vi "AMI 430_Hardware_Module_X AXIS.vi"(5 "Enable":bool=TRUE, 7 "Command":T4, 8 "error in (no error)":errorcluster, 9 "Settings":T2={"magneticFieldUnits"=1, "rampRateUnits"=1, "rampRate"=0.0, "targetField"=0.0, "rampingMode"=1} {"rampingMode" items=["RAMP", "PAUSE", "MANUAL UP", "MANUAL DOWN", "ZERO"]; "targetField" format="%.4f"; "rampRate" format="%.1f"; "rampRateUnits" items=["Per SECOND", "Per MINUTE"]; "magneticFieldUnits" items=["KGauss", "Tesla"]}, 11 "Comm Config In":T3={"connection ID"=refnum, "IP"="192.168.0.108", "Active Comm Interface"=0, "Serial Port"="", "Programmer Type"=0, "connection ID"=refnum, "output cluster"={"GPIB address"=22, "GPIB bus"=1}} caption="X AXIS: 192.168.0.108" {"Programmer Type" items=["Model 430", "Model 420"]; "Active Comm Interface" items=["TCP/IP (Model 430 Only)", "RS232", "IEEE488"]}) -> (0 "error out":errorcluster, 1 "magneticField":dbl format="%.6f", 2 "Instrument Responded?":bool, 3 "Comm Config Out":T3={"connection ID"=refnum, "IP"="192.168.0.108", "Active Comm Interface"=0, "Serial Port"="", "Programmer Type"=0, "connection ID"=refnum, "output cluster"={"GPIB address"=22, "GPIB bus"=1}} {"Programmer Type" items=["Model 430", "Model 420"]; "Active Comm Interface" items=["TCP/IP (Model 430 Only)", "RS232", "IEEE488"]}, 4 "state":T1=1 items=["Unknown", "RAMPING to target field/current", "HOLDING at the target field/current", "PAUSED", "Ramping in MANUAL UP mode", "Ramping in MANUAL DOWN mode", "ZEROING CURRENT (in progress)", "Quench detected", "At ZERO current", "Heating persistent switch", "Cooling persistent switch", "External Rampdown active"])   [LabVIEW 2017]
uses:
  AMI 430_Hardware_Module.ctl
  commsControl.ctl
  magneticField.ctl
  Status AMI.ctl
panel:
  # "X AXIS"
  # "AMI 430 MAGNETIC FIELD SYSTEM"
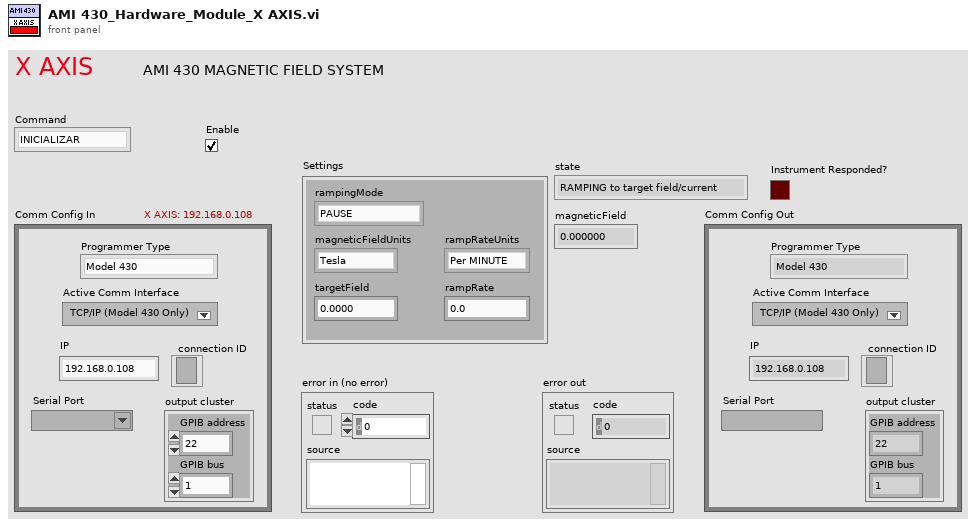
[diagram p1: front panel]
types:
  T1 = typedef "Status AMI.ctl" = u16
  T2 = typedef "magneticField.ctl" = cluster{"magneticFieldUnits":u16, "rampRateUnits":u16, "rampRate":dbl, "targetField":dbl, "rampingMode":u16}
  T3 = typedef "commsControl.ctl" = cluster{"connection ID":refnum<k5>, "IP":string, "Active Comm Interface":u16, "Serial Port":refnum<visa-resource-name>, "Programmer Type":u16, "connection ID":refnum<k5>, "output cluster":cluster{"GPIB address":i16, "GPIB bus":i16}}
  T4 = typedef "AMI 430_Hardware_Module.ctl" = enum16{"INICIALIZAR", "SET UNIDADES CAMPO", "SET UNIDADES RAMPA", "SET CAMPO", "SET  RAMPA", "SET RAMPING MODE", "READ CAMPO", "STATUS", "SHUTDOWN"}
  T5 = cluster{"error":bool, "code":i32, "source":string}
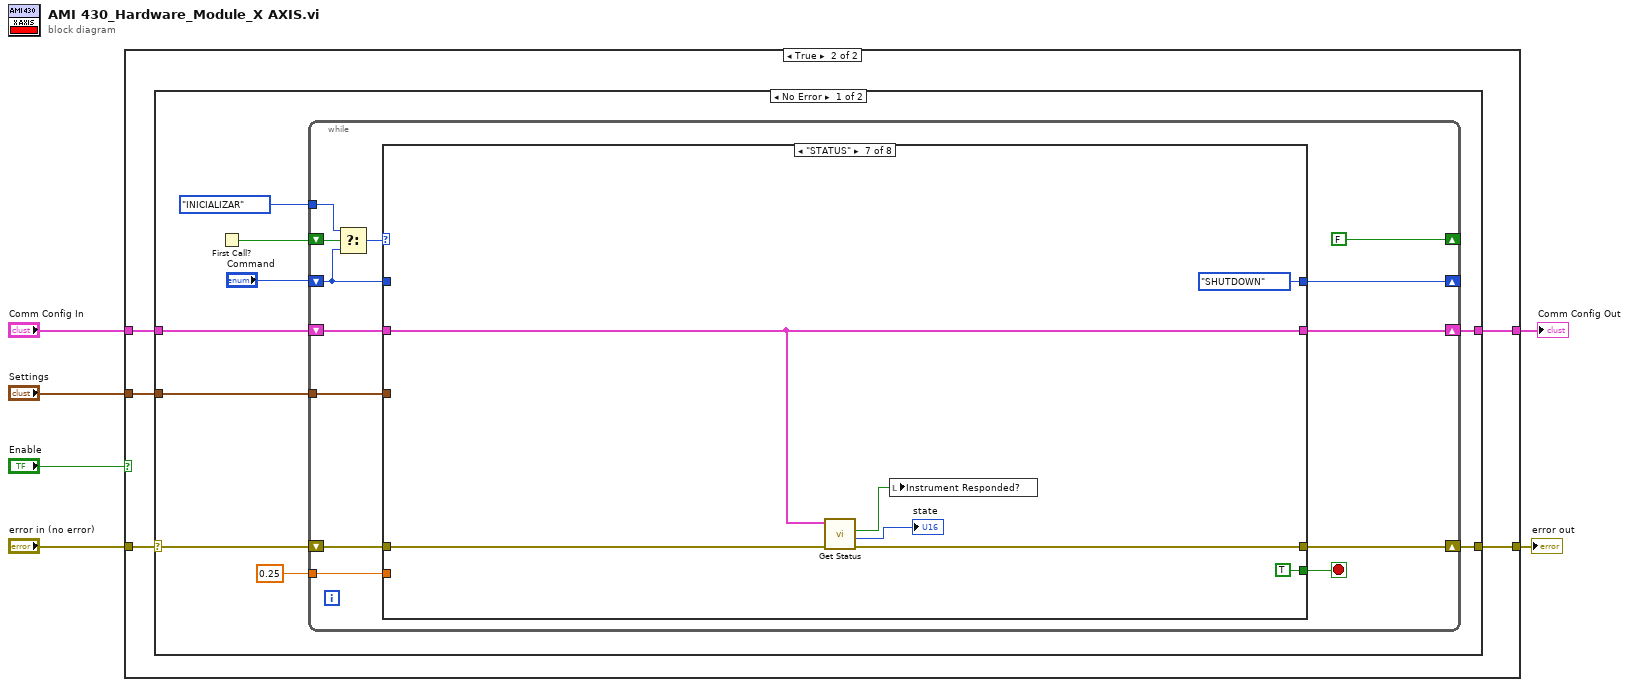
[diagram p0: block diagram]
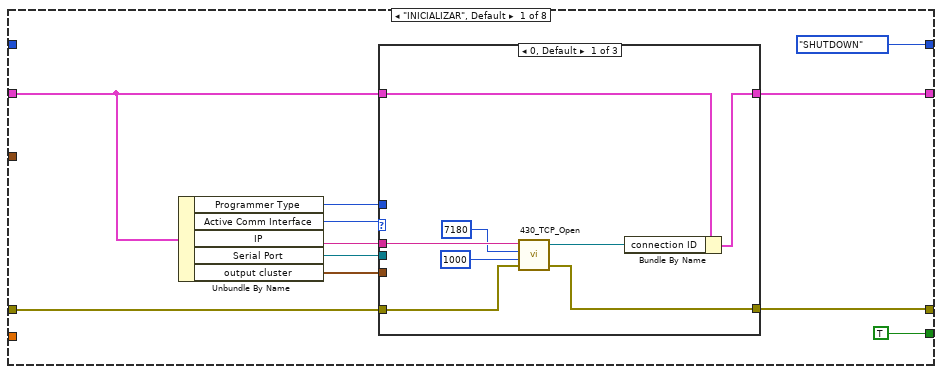
[diagram p3: hidden frame]
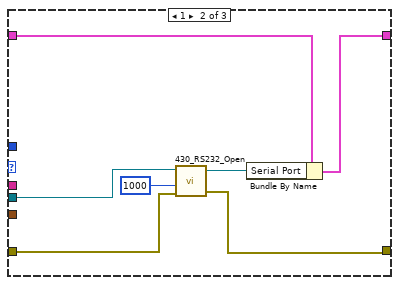
[diagram p4: hidden frame]
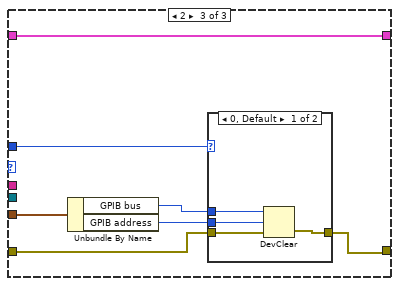
[diagram p5: hidden frame]
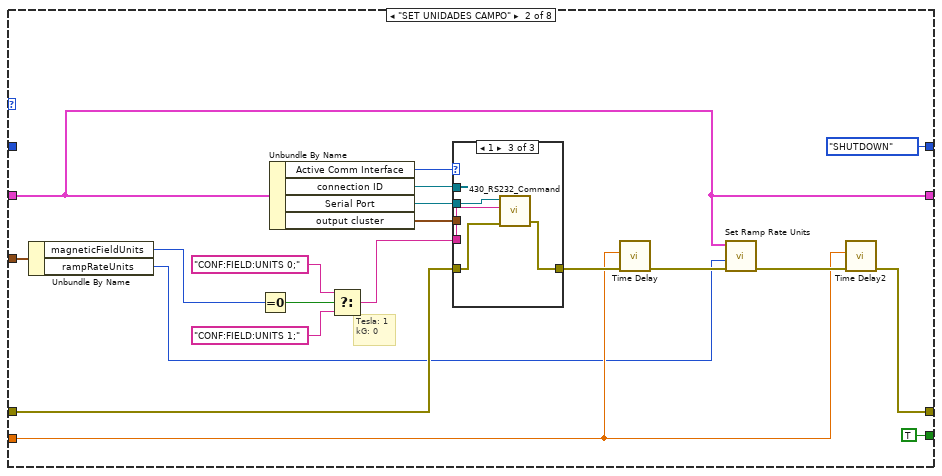
[diagram p7: hidden frame]
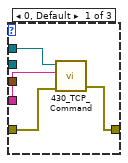
[diagram p8: hidden frame]
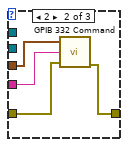
[diagram p9: hidden frame]
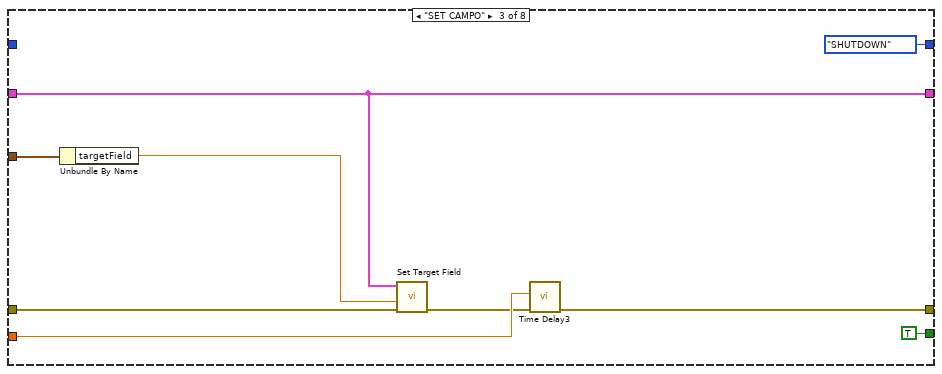
[diagram p10: hidden frame]
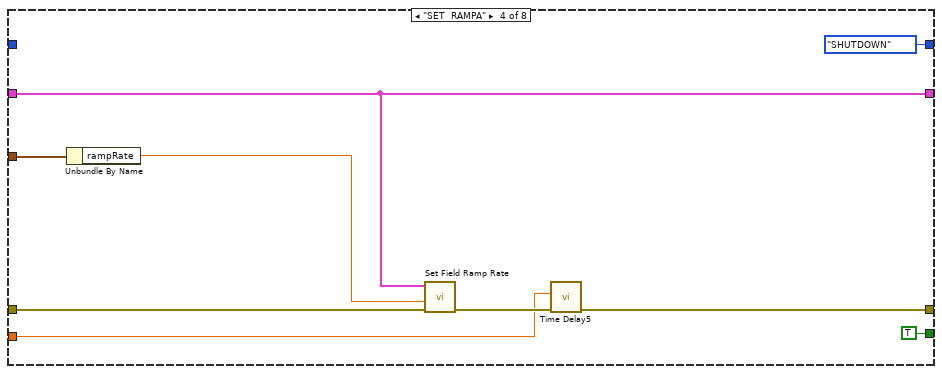
[diagram p11: hidden frame]
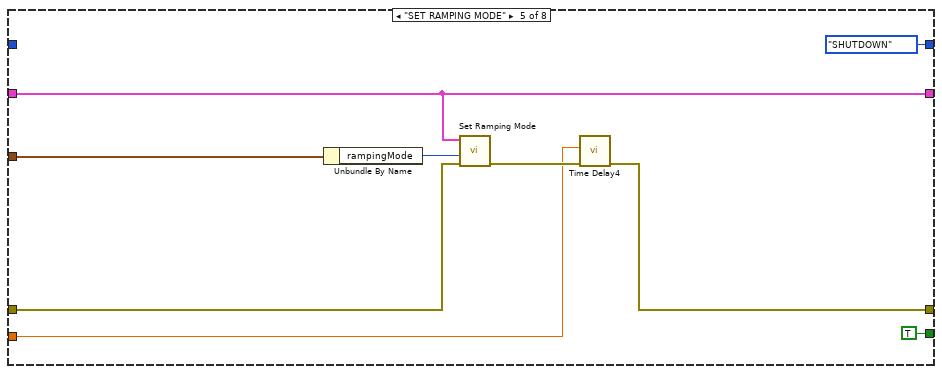
[diagram p12: hidden frame]
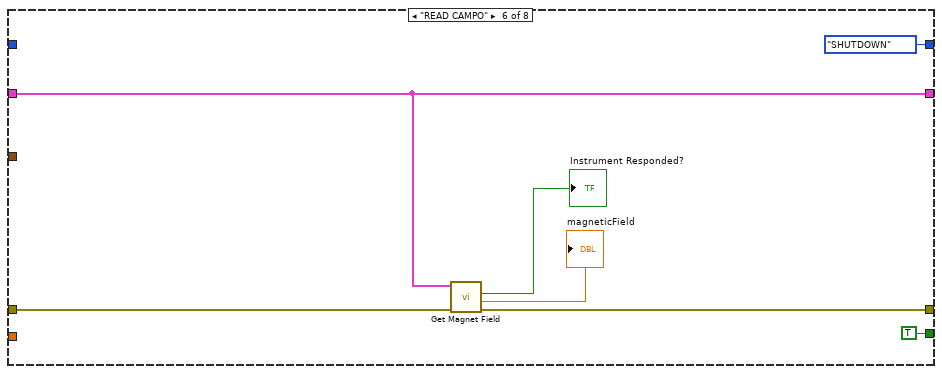
[diagram p13: hidden frame]
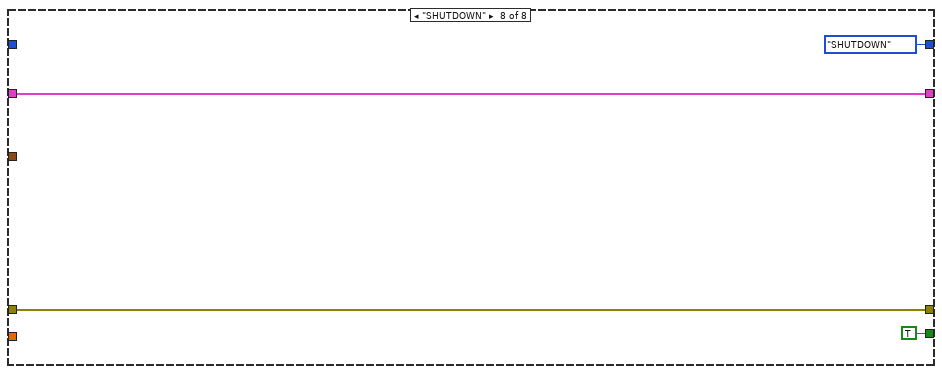
[diagram p14: hidden frame]
diagram:
  n1 = case shown="True" "Enable" {
    tunnel: "error in (no error)" -> [w8 w13]
    tunnel: [w8 w12] -> w5
    tunnel: "Comm Config In" -> [w7 w11]
    tunnel: [w7 w10] -> w2
    tunnel: "Settings" -> [_ w9]
    frame False {
    }
    frame True {
      n2 = case shown="No Error" w13 {
        selector: w13 -> [w20 w152]
        tunnel: [w19 w152] -> w12
        tunnel: w11 -> [w17 w151]
        tunnel: [w16 w151] -> w10
        tunnel: w9 -> [w15 _]
        frame No Error {
          n3 = First Call?() -> (First Call?: T/F=w22:bool)
          n4 = while {
            shift-right: [w30] -> _
            shift-left: "Command" -> [w31]
            shift-right: [w28] -> w19
            shift-left: w20 -> [w26]
            shift-right: [FALSE ("First Call?: T/F")] -> _
            shift-left: w22 -> [w35]
            tunnel: AMI_430_Hardware_Module."INICIALIZAR" ("t") -> [w34]
            shift-right: [w25] -> w16
            shift-left: w17 -> [w27]
            tunnel: w15 -> [w24]
            tunnel: 0.25 ("Delay Time (s)") -> [w23]
            stop <- w29 stop-if-true
            n5 = Select(t=w34, s=w35, f=w31) -> (s? t:f=w32:T4)
            n6 = case shown="\"STATUS\"" w32 {
              tunnel: w31 -> [_ _ _ _ _ _ _ _]
              tunnel: [AMI_430_Hardware_Module."SHUTDOWN" ("s? t:f") AMI_430_Hardware_Module."SHUTDOWN" ("s? t:f") AMI_430_Hardware_Module."SHUTDOWN" ("s? t:f") AMI_430_Hardware_Module."SHUTDOWN" ("s? t:f") AMI_430_Hardware_Module."SHUTDOWN" ("s? t:f") AMI_430_Hardware_Module."SHUTDOWN" ("s? t:f") AMI_430_Hardware_Module."SHUTDOWN" ("s? t:f") AMI_430_Hardware_Module."SHUTDOWN" ("s? t:f")] -> w30
              tunnel: [TRUE ("First Call?: T/F") TRUE ("First Call?: T/F") TRUE ("First Call?: T/F") TRUE ("First Call?: T/F") TRUE ("First Call?: T/F") TRUE ("First Call?: T/F") TRUE ("First Call?: T/F") TRUE ("First Call?: T/F")] -> w29
              tunnel: [w39 w76 w112 w120 w130 w138 w145 w150] -> w28
              tunnel: w27 -> [w38 w87 w109 w117 w125 w135 w142 w147]
              tunnel: [w37 w87 w109 w117 w125 w135 w142 w147] -> w25
              tunnel: w26 -> [w36 w88 w106 w121 w132 w139 w146 w150]
              tunnel: w24 -> [_ w79 w108 w116 w128 _ _ _]
              tunnel: w23 -> [_ w75 w114 w122 w129 _ _ _]
              frame "INICIALIZAR", Default {
                n7 = Unbundle By Name(w38) -> ("Programmer Type"=w40:u16, "Active Comm Interface"=w42:u16, "IP"=w44:string, "Serial Port"=w43:refnum<visa-resource-name>, "output cluster"=w41:cluster{"GPIB address":i16, "GPIB bus":i16})
                n8 = case shown="0, Default" w42 {
                  tunnel: w38 -> [w54 w59 w65]
                  tunnel: w36 -> [w52 w60 w68]
                  tunnel: [w51 w57 w67] -> w39
                  tunnel: w44 -> [w50 _ _]
                  tunnel: [w47 w58 w65] -> w37
                  tunnel: w43 -> [_ w56 _]
                  tunnel: w41 -> [_ _ w64]
                  tunnel: w40 -> [_ _ w66]
                  frame 0, Default {
                    n9 = call "430_TCP_Open.vi"("IP Address"=w50, "TCP Port"=7180, "timeout ms (2000)"=1000 ("timeout ms (60000)"), "error in (no error)"=w52) -> ("connection ID"=w53:refnum<k5>, "error out"=w51:errorcluster)  [unwired: 2 in, 1 out]
                    n10 = Bundle By Name(cluster=w54, "connection ID"=w53) -> (w47:T3)
                  }
                  frame 1 {
                    n11 = call "430_RS232_Open.vi"("VISA resource name"=w56, "timeout ms (2000)"=1000 ("timeout ms (60000)"), "error in (no error)"=w60) -> ("VISA resource name out"=w61:refnum<visa-resource-name>, "error out"=w57:errorcluster)  [unwired: 4 in]
                    n12 = Bundle By Name(cluster=w59, "Serial Port"=w61) -> (w58:T3)
                  }
                  frame 2 {
                    n13 = Unbundle By Name(w64) -> ("GPIB bus"=w63:i16, "GPIB address"=w62:i16)
                    n14 = case shown="0, Default" w66 {
                      tunnel: w68 -> [w72 w73]
                      tunnel: [w71 w73] -> w67
                      tunnel: w63 -> [w70 _]
                      tunnel: w62 -> [w69 _]
                      frame 0, Default {
                        n15 = DevClear(2:w72, 3:w69, 4:w70) -> (0:w71:errorcluster)  [unwired: 1 out]
                      }
                      frame 1 {
                      }
                    }
                  }
                }
              }
              frame "SET UNIDADES CAMPO" {
                # "Tesla: 1\nkG: 0"
                n16 = Unbundle By Name(w79) -> ("magneticFieldUnits"=w78:u16, "rampRateUnits"=w74:u16)
                n17 = Equal To 0?(x=w78) -> (x = 0?=w81:bool)
                n18 = Unbundle By Name(w87) -> ("Active Comm Interface"=w93:u16, "connection ID"=w92:refnum<k5>, "Serial Port"=w91:refnum<visa-resource-name>, "output cluster"=w86:cluster{"GPIB address":i16, "GPIB bus":i16})
                n19 = Select(t="CONF:FIELD:UNITS 0;", s=w81, f="CONF:FIELD:UNITS 1;") -> (s? t:f=w80:string)
                n20 = case shown="1" w93 {
                  tunnel: w92 -> [w97 _ _]
                  tunnel: w80 -> [w96 w101 w104]
                  tunnel: w88 -> [w95 w99 w103]
                  tunnel: w86 -> [_ w100 _]
                  tunnel: w91 -> [_ _ w105]
                  tunnel: [w94 w98 w102] -> w85
                  frame 0, Default {
                    n21 = call "430_TCP_Command.vi"("error in (no error)"=w95, "Command"=w96, "connection ID"=w97) -> ("error out"=w94:errorcluster)  [unwired: 1 in, 2 out]
                  }
                  frame 2 {
                    n22 = call "GPIB 332 Command.vi"("GPIB (In)"=w100, "Input command"=w101, "error in"=w99) -> ("error out"=w98:T5)  [unwired: 3 out]
                  }
                  frame 1 {
                    n23 = call "430_RS232_Command.vi"("error in (no error)"=w103, "Command"=w104, "VISA resource name"=w105) -> ("error out"=w102:errorcluster)  [unwired: 1 in, 2 out]
                  }
                }
                n24 = call "Time Delay"("error in (no error)"=w85, "Delay Time (s)"=w75) -> ("error out"=w84:errorcluster)  [unwired: 9 in]
                n25 = call "Set Ramp Rate Units.vi"("error in"=w84, "Ramp Rate Units"=w74, "Communications Config"=w87) -> ("error out"=w77:T5)  [unwired: 8 in]
                n26 = call "Time Delay2"("error in (no error)"=w77, "Delay Time (s)"=w75) -> ("error out"=w76:errorcluster)  [unwired: 9 in]
              }
              frame "SET CAMPO" {
                n27 = Unbundle By Name(w108) -> ("targetField"=w107:dbl)
                n28 = call "Set Target Field.vi"("error in"=w106, "Target Field (kG)"=w107, "Communications Config"=w109) -> ("error out"=w113:T5)  [unwired: 8 in]
                n29 = call "Time Delay3"("error in (no error)"=w113, "Delay Time (s)"=w114) -> ("error out"=w112:errorcluster)  [unwired: 9 in]
              }
              frame "SET  RAMPA" {
                n30 = Unbundle By Name(w116) -> ("rampRate"=w115:dbl)
                n31 = call "Set Field Ramp Rate.vi"("error in"=w121, "Ramp Rate (kG/sec)"=w115, "Communications Config"=w117) -> ("error out"=w123:T5)  [unwired: 8 in]
                n32 = call "Time Delay5"("error in (no error)"=w123, "Delay Time (s)"=w122) -> ("error out"=w120:errorcluster)  [unwired: 9 in]
              }
              frame "SET RAMPING MODE" {
                n33 = Unbundle By Name(w128) -> ("rampingMode"=w127:u16)
                n34 = call "Set Ramping Mode.vi"("error in"=w132, "Ramping Mode"=w127, "Communications Config"=w125) -> ("error out"=w131:T5)  [unwired: 8 in]
                n35 = call "Time Delay4"("error in (no error)"=w131, "Delay Time (s)"=w129) -> ("error out"=w130:errorcluster)  [unwired: 9 in]
              }
              frame "READ CAMPO" {
                n36 = call "Get Magnet Field.vi"("error in"=w139, "Communications Config"=w135) -> ("error out"=w138:T5, "Magnet Field (kG)"=→"magneticField":dbl, "Instrument Responded?"=→"Instrument Responded?":bool)  [unwired: 7 in]
              }
              frame "STATUS" {
                n37 = call "Get Status.vi"("error in"=w146, "Communications Config"=w142) -> ("error out"=w145:T5, "state"=→"state":T1, "Instrument Responded?"=w140:bool)  [unwired: 7 in]
                n38 = local write "Instrument Responded?"(w140) -> ()
              }
              frame "SHUTDOWN" {
              }
            }
          }
        }
        frame Error {
        }
      }
    }
  }
  "error out" <- w5
  "Comm Config Out" <- w2
